vi "Scalar Inputs.vi"(8 "error in (no error)":errorcluster, 11 "Node Ptr":T1 format="%.0x") -> (0 "error out":errorcluster)   [LabVIEW 2016, in "FPGA Addon System Explorer.lvlib"]
uses:
  FPGA Addon System Explorer.lvlib
  <vilib>/NI Veristand/Custom Device API/Custom Device Item Ref.ctl
  FPGA-Resource-Manager-APIs/Source/Shared/Types/Channel Type.ctl
  FPGA-Resource-Manager-APIs/Source/System Definition/API/Server-Specific/Resource Groups/get fpga resources compatible with FPGA Addon CD group.vi
  FPGA-Resource-Manager-APIs/Source/Shared/find Relative VS Ref.vi
  FPGA-Resource-Manager-APIs/Source/System Definition/API/FPGA Resource Discovery/get FPGA resources for this FPGA Addon CD.vi
  SubVIs/RegMap to Register Information.vi
  <vilib>/NI VeriStand/Custom Device API/Custom Device API.lvlib
  FPGA-Resource-Manager-APIs/Source/Shared/FPGA RM Shared API.lvlib
panel:
  in  "remove":bool
  in  "add":bool
  in  "Available Registers":i32[](listbox)
  in  "Header 2":cluster{"Section Name":string}={"Section Name"="Custom Device Item Settings"}
  in  "SHDocVw.IWebBrowser":refnum<k7>(container)
  in  "Header":cluster{"Section Name":string}={"Section Name"="Custom Device Item Settings"}
  in  "Description":string
  out "Name":string
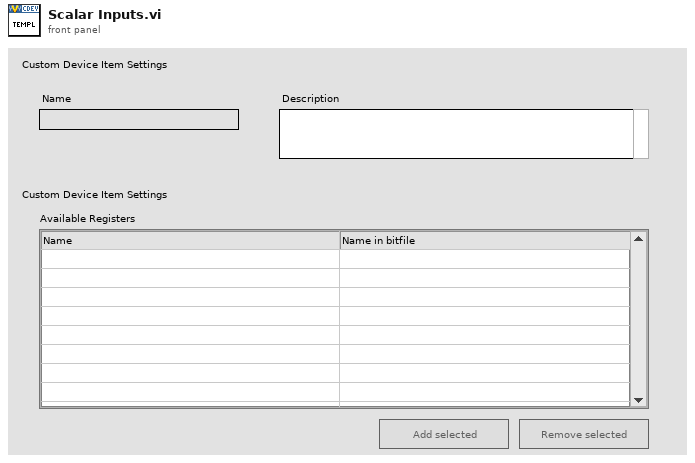
[diagram p1: front panel]
types:
  T1 = typedef "Custom Device API.lvlib/Custom Device Item Ref.ctl" = u64
  T2 = typedef "Custom Device API.lvlib/Custom Device Item Info.ctl" = cluster{"Name":string, "Is Channel":bool, "GUID":string, "Is Waveform":bool}
  T3 = typedef "FPGA RM Shared API.lvlib/Register Information.ctl" = cluster{"Name":string, "Data Type":T4, "Default Value":variant}
  T4 = typedef "FPGA RM Shared API.lvlib/Data Type.ctl" = enum8{"<Null>", "I8", "I16", "I32", "I64", "U8", "U16", "U32", "U64", "SGL", "Boolean", "Analog PWM In Settings", "Analog PWM In", "Digital PWM In Settings", "Digital PWM In", "Digital PWM Out", "Sine Out", "FXP+/-24.5", "FXP+/-16.5", "FXP+/-32.8", "FXP+/-64.32", "FXP+/-16.7", "FXP+/-20.5"}
  T5 = typedef "FPGA Addon System Explorer.lvlib/Listbox Cluster.ctl" = cluster{"add":refnum<vi>, "remove":refnum<vi>, "Listbox":refnum<vi>, "selected":i32[], "not present":i32[], "reserved":i32[], "listbox text":string[][], "Section Ref":T1}
  T6 = typedef "FPGA RM Shared API.lvlib/Channel Type.ctl" = enum16{"Write Channel", "Read Channel", "Write Waveform", "Read Waveform"}
  T7 = typedef "Custom Device API.lvlib/Custom Device Commands.ctl" = enum16{"Default", "Item renamed", "Shutdown", "Dynamic button pressed"}
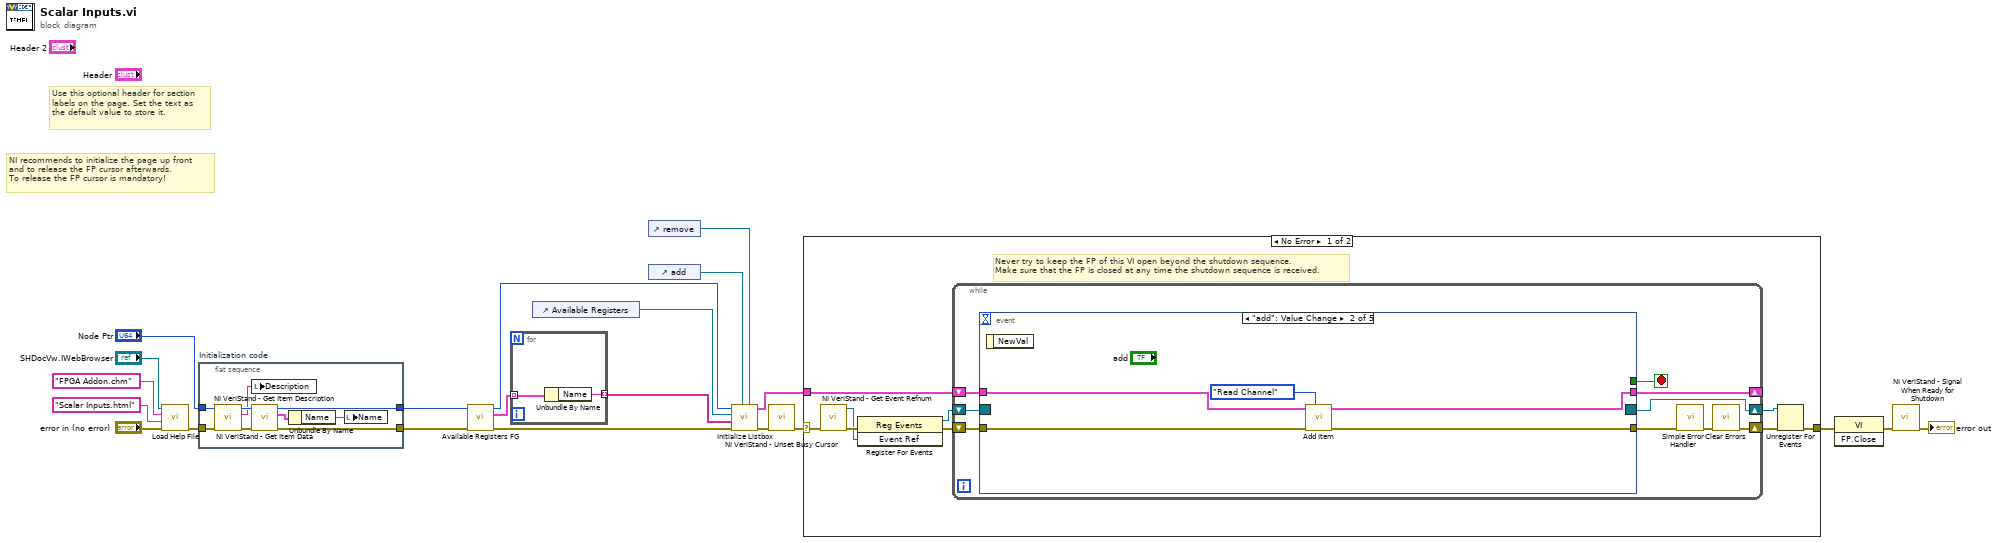
[diagram p0: block diagram]
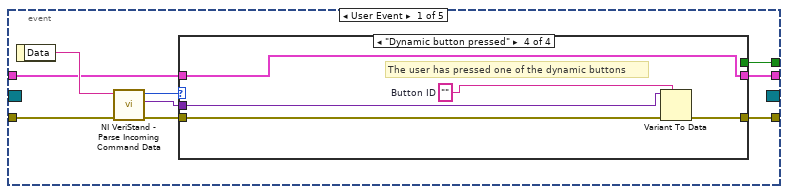
[diagram p2: hidden frame]
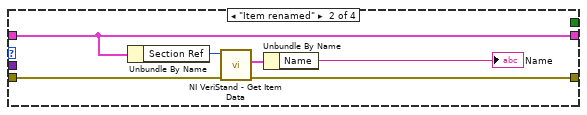
[diagram p4: hidden frame]
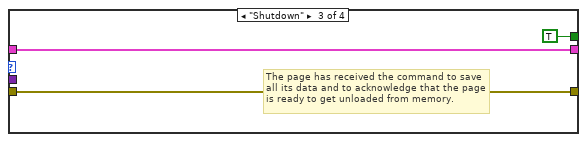
[diagram p5: hidden frame]
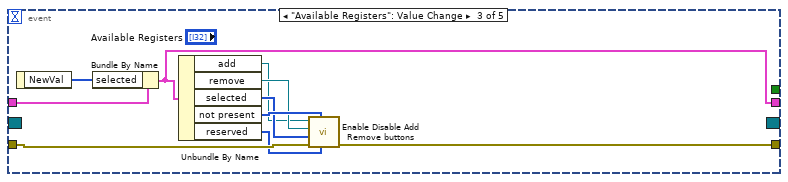
[diagram p6: hidden frame]
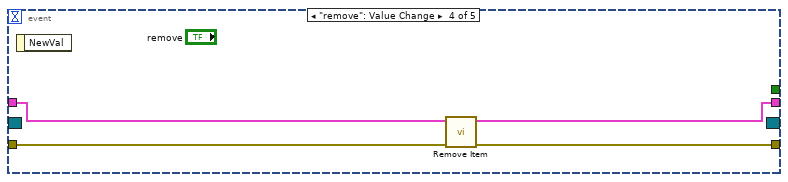
[diagram p7: hidden frame]
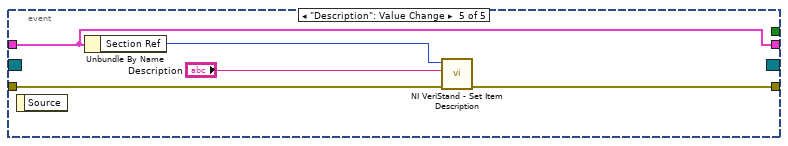
[diagram p8: hidden frame]
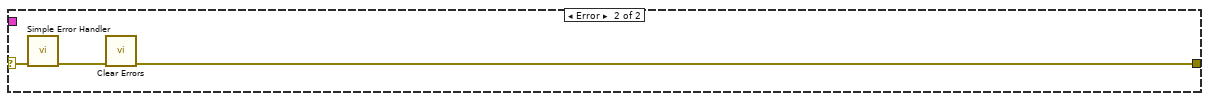
[diagram p9: hidden frame]
diagram:
  # "Use this optional header for section labels on the page. Set the text as the default value to store it."
  # "NI recommends to initialize the page up front\nand to release the FP cursor afterwards.\nTo release the FP cursor is mandatory!"
  n1 = call "Load Help File.vi"("error in (no error)"="error in (no error)", "HTML File"="Scalar Inputs.html", "Main CHM File"="FPGA Addon.chm", "SHDocVw.IWebBrowser2"="SHDocVw.IWebBrowser") -> ("error out"=w12:errorcluster)  [unwired: 7 in]
  n2 = flat-sequence "Initialization code" {
    tunnel: w12 -> [w28]
    tunnel: "Node Ptr" -> [w27]
    tunnel: [w22] -> w11
    tunnel: [w30] -> w10
    frame #0 {
      n3 = call <vilib>:"NI VeriStand - Get Item Description.vi"("error in (no error)"=w28, "Item Ref in"=w27) -> ("error out"=w25:errorcluster, "Description"=w26:string, "Item Ref out"=w29:T1)  [unwired: 7 out]
      n4 = local write "Description"(w26) -> ()
      n5 = call <vilib>:"NI VeriStand - Get Item Data.vi"("error in (no error)"=w25, "Item Ref in"=w29) -> ("error out"=w22:errorcluster, "Item Info"=w24:T2, "Item Ref out"=w30:T1)  [unwired: 7 out]
      n6 = Unbundle By Name(w24) -> ("Name"=w23:string)
      n7 = local write "Name"(w23) -> ()
    }
  }
  n8 = call "Available Registers FG.vi"("error in (no error)"=w11, "Item Ref"=w10) -> ("error out"=w8:errorcluster, "Available Registers"=w9:T3[], "Item Ref out"=w2:T1)  [unwired: 7 in]
  n9 = for {
    tunnel: w9 -> [w32] mode=indexing
    tunnel: [w31] -> w7 mode=indexing
    n10 = Unbundle By Name(w32) -> ("Name"=w31:string)
  }
  n11 = control-ref of="Available Registers"() -> (w6:refnum<vi>)
  n12 = control-ref of="remove"() -> (w4:refnum<vi>)
  n13 = control-ref of="add"() -> (w5:refnum<vi>)
  n14 = call "Initialize Listbox.vi"("remove"=w4, "add"=w5, "error in (no error)"=w8, "Names"=w7, "Listbox"=w6, "Item Ref"=w2) -> ("error out"=w3:errorcluster, "Listbox Refs"=w1:T5)  [unwired: 4 in]
  n15 = call <vilib>:"NI VeriStand - Unset Busy Cursor.vi"("error in (no error)"=w3) -> ("error out"=w17:errorcluster)  [unwired: 10 out]
  n16 = case shown="No Error" w17 {
    selector: w17 -> [w34 w102]
    tunnel: [w38 w100] -> w21
    tunnel: w1 -> [w33 _]
    frame No Error {
      # "Never try to keep the FP of this VI open beyond the shutdown sequence.\nMake sure that the FP is closed at any time the shutdown sequence is received."
      n17 = call <vilib>:"NI VeriStand - Get Event Refnum.vi"("error in (no error)"=w34) -> ("error out"=w41:errorcluster, "Event Ref"=w37:refnum<user-event>)  [unwired: 9 out]
      n18 = register-events(error in=w41, w37) -> (reference out=w35:refnum<event-registration>, error out=w36:errorcluster)  [unwired: 1 in]
      n19 = while {
        shift-right: [w44] -> w39
        shift-left: w36 -> [w49]
        shift-right: [w50] -> w40
        shift-left: w35 -> [w48]
        shift-right: [w42] -> _
        shift-left: w33 -> [w43]
        stop <- w47 stop-if-true
        n20 = event shown="[1] \"add\": Value Change" {
          selector: w48 -> [_ _ _ _ _]
          dyn-events: [_ _ _ _ _] -> w50
          timeout: _ -> [_ _ _ _ _]
          tunnel: w49 -> [w59 w80 w90 w93 w99]
          tunnel: [w55 _ _ _ _] -> w47
          tunnel: [w54 w79 w89 w94 w98] -> w46
          tunnel: w43 -> [w52 w77 w87 w92 w96]
          tunnel: [w51 w78 w86 w91 w96] -> w42
          event User Event {
            n21 = event-data() -> ("Data"=w58:string)  [unwired: 1 out]
            n22 = call <vilib>:"NI VeriStand - Parse Incoming Command Data.vi"("error in (no error)"=w59, "Incoming data"=w58) -> ("error out"=w57:errorcluster, "Outgoing data"=w53:variant, "Action"=w56:T7)  [unwired: 7 out]
            n23 = case shown="\"Dynamic button pressed\"" w56 {
              tunnel: w57 -> [w61 w67 w69 w75]
              tunnel: [_ _ TRUE _] -> w55
              tunnel: [w61 w65 w69 w72] -> w54
              tunnel: w53 -> [_ _ _ w74]
              tunnel: w52 -> [w60 w63 w68 w71]
              tunnel: [w60 w63 w68 w71] -> w51
              frame "Default", Default {
              }
              frame "Item renamed" {
                n24 = Unbundle By Name(w63) -> ("Section Ref"=w64:T1)
                n25 = call <vilib>:"NI VeriStand - Get Item Data.vi"("error in (no error)"=w67, "Item Ref in"=w64) -> ("error out"=w65:errorcluster, "Item Info"=w66:T2)  [unwired: 8 out]
                n26 = Unbundle By Name(w66) -> ("Name"=→"Name":string)
              }
              frame "Shutdown" {
                # "The page has received the command to save all its data and to acknowledge that the page is ready to get unloaded from memory."
              }
              frame "Dynamic button pressed" {
                w73 = ""  # Button ID
                # "The user has pressed one of the dynamic buttons"
                n27 = Variant To Data(error in=w75, type=w73, Variant=w74) -> (error out=w72:errorcluster)  [unwired: 1 out]
              }
            }
          }
          event "add": Value Change {
            n28 = event-data() -> ()  [unwired: 2 out]
            n29 = call "Add Item.vi"("Action"=Channel_Type."Read Channel", "error in (no error)"=w80, "Listbox Refs in"=w77) -> ("error out"=w79:errorcluster, "Listbox Refs out"=w78:T5)  [unwired: 7 in]
          }
          event "Available Registers": Value Change {
            n30 = event-data() -> ("NewVal"=w85:i32[])  [unwired: 1 out]
            n31 = Bundle By Name(cluster=w87, "selected"=w85) -> (w86:T5)
            n32 = Unbundle By Name(w86) -> ("add"=w82:refnum<vi>, "remove"=w83:refnum<vi>, "selected"=w84:i32[], "not present"=w88:i32[], "reserved"=w81:i32[])
            n33 = call "Enable Disable Add Remove buttons.vi"("reserved item indexes"=w81, "not present item indexes"=w88, "error in (no error)"=w90, "selected items"=w84, "remove button"=w83, "add button"=w82) -> ("error out"=w89:errorcluster)  [unwired: 5 in]
          }
          event "remove": Value Change {
            n34 = event-data() -> ()  [unwired: 2 out]
            n35 = call "Remove Item.vi"("error in (no error)"=w93, "Listbox Refs in"=w92) -> ("error out"=w94:errorcluster, "Listbox Refs out"=w91:T5)  [unwired: 8 in]
          }
          event "Description": Value Change {
            n36 = event-data() -> ()  [unwired: 2 out]
            n37 = Unbundle By Name(w96) -> ("Section Ref"=w95:T1)
            n38 = call <vilib>:"NI VeriStand - Set Item Description.vi"("error in (no error)"=w99, "Description"="Description", "Item Ref in"=w95) -> ("error out"=w98:errorcluster)  [unwired: 8 out]
          }
        }
        n39 = call <vilib>:"Simple Error Handler.vi"("error in (no error)"=w46) -> ("error out"=w45:errorcluster)  [unwired: 1 in, 7 out]
        n40 = call <vilib>:"Clear Errors.vi"("error in (no error)"=w45) -> ("error out"=w44:errorcluster)  [unwired: 1 in, 5 out]
      }
      n41 = Unregister For Events(event registration refnum=w40, error in=w39) -> (error out=w38:errorcluster)
    }
    frame Error {
      n42 = call <vilib>:"Simple Error Handler.vi"("error in (no error)"=w102) -> ("error out"=w101:errorcluster)  [unwired: 1 in, 7 out]
      n43 = call <vilib>:"Clear Errors.vi"("error in (no error)"=w101) -> ("error out"=w100:errorcluster)  [unwired: 1 in, 5 out]
    }
  }
  n44 = invoke class="VI" method="FP.Close"(error in=w21) -> (error out=w20:errorcluster)  [unwired: 2 in, 2 out]
  n45 = call <vilib>:"NI VeriStand - Signal When Ready for Shutdown.vi"("error in (no error)"=w20) -> ("error out"=→"error out":errorcluster)  [unwired: 10 out]
